vi "Write Length Value.vi"(8 "error in (no error)":errorcluster, 10 "Length (auto)":string, 11 "Element Array in":refnum<class "Element Array.lvclass">) -> (0 "error out":errorcluster, 3 "Element Array out":refnum<class "Element Array.lvclass">)   [LabVIEW 2023, in "VILab.lvlib" / "Element Array.lvclass"]
uses:
  Element Array.lvclass
  Element Array.lvclass/Element Array.ctl
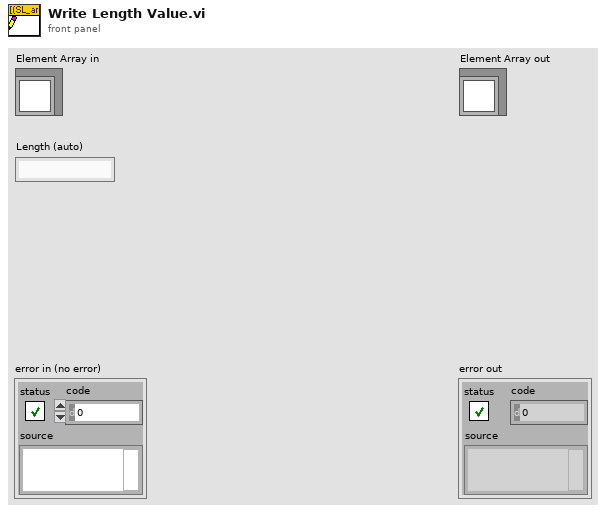
[diagram p1: front panel]
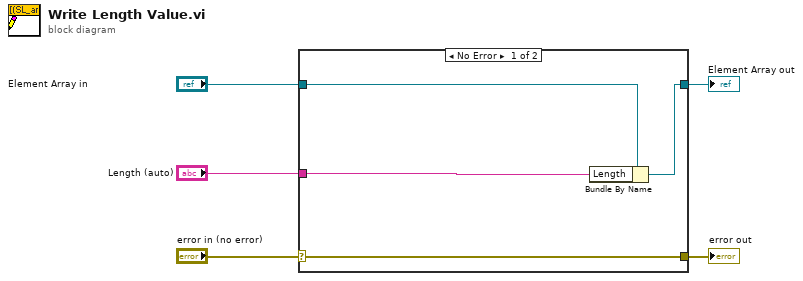
[diagram p0: block diagram]
diagram:
  n1 = case shown="No Error" "error in (no error)" {
    selector: "error in (no error)" -> [w9 w10]
    tunnel: [w9 w10] -> w4
    tunnel: [w7 w11] -> w2
    tunnel: "Element Array in" -> [w8 w11]
    tunnel: "Length (auto)" -> [w6 _]
    frame No Error {
      n2 = Bundle By Name(cluster=w8, "Length"=w6) -> (w7:refnum<class "Element Array.lvclass">)
    }
    frame Error {
    }
  }
  "error out" <- w4
  "Element Array out" <- w2
